vi "Out_S6F11.vi"(8 "error in (no error)":errorcluster, 10 "S6F11":T1, 11 "S6 Message Class in":refnum<class "S6 Message Class.lvclass">) -> (0 "error out":errorcluster, 3 "S6 Message Class out":refnum<class "S6 Message Class.lvclass">)   [LabVIEW 2020, in "SECS Communication.lvlib" / "S6 Message Class.lvclass"]
uses:
  S6 Message Class.lvclass
  D:/Dropbox/SECS/SECS_GEM v1.0.6/Com/SECS Communication/SECS-II Class/SECS-II Class.lvclass
  S6F11.ctl
  SECS-II Class/Format Code.ctl
  SECS-II Class/Data Message_List.vi
  SECS-II Class/Data Message_U4.vi
  SECS-II Class/Variant To Data_ASCII.vi
  SECS-II Class/Data Message_ASCII.vi
  SECS-II Class/Variant To Data_Binary.vi
  SECS-II Class/Data Message_Binary.vi
  SECS-II Class/Variant To Data_Boolean.vi
  SECS-II Class/Data Message_Boolean.vi
  SECS-II Class/Variant To Data_J.vi
  SECS-II Class/Data Message_J.vi
  SECS-II Class/Variant To Data_I1.vi
  SECS-II Class/Data Message_I1 .vi
  SECS-II Class/Variant To Data_I2.vi
  SECS-II Class/Data Message_I2.vi
  SECS-II Class/Variant To Data_I4.vi
  SECS-II Class/Data Message_I4.vi
  SECS-II Class/Variant To Data_I8.vi
  SECS-II Class/Data Message_I8.vi
  SECS-II Class/Variant To Data_U1.vi
  SECS-II Class/Data Message_U1.vi
  SECS-II Class/Variant To Data_U2.vi
  SECS-II Class/Data Message_U2.vi
  SECS-II Class/Variant To Data_U4.vi
  SECS-II Class/Variant To Data_U8.vi
  SECS-II Class/Data Message_U8.vi
  SECS-II Class/Variant To Data_F4.vi
  SECS-II Class/Data Message_F4.vi
  SECS-II Class/Variant To Data_F8.vi
  SECS-II Class/Data Message_F8.vi
  SECS-II Class/Variant To Data_Character.vi
  SECS-II Class/Data Message_Character.vi
  SECS-II Class/SECS-II Class.lvclass
  D:/Dropbox/SECS/SECS_GEM v1.0.6/Com/SECS Communication/S6 Message Class/S6 Message Class.lvclass
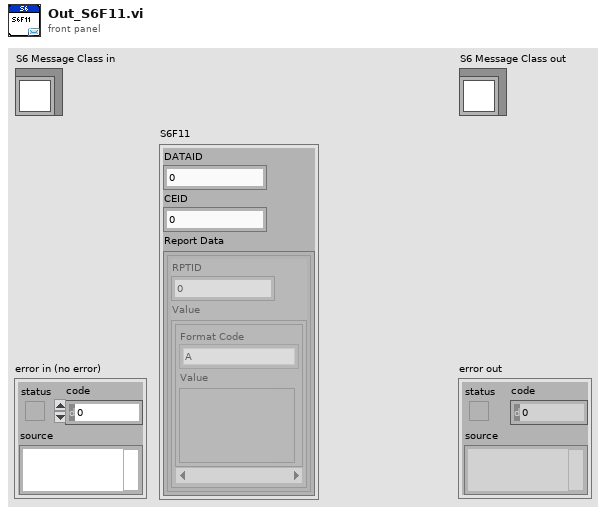
[diagram p1: front panel]
types:
  T1 = typedef "SECS Communication.lvlib/S6 Message Class.lvclass/S6F11.ctl" = cluster{"DATAID":u32, "CEID":u32, "Report Data":cluster{"RPTID":u32, "Value":cluster{"Format Code":T2, "Value":variant}[]}[]}
  T2 = typedef "SECS Communication.lvlib/SECS-II Class.lvclass/Format Code.ctl" = enum16{"L", "A", "B", "Boolean", "J", "I1", "I2", "I4", "I8", "U1", "U2", "U4", "U8", "F4", "F8", "Char"}
  T3 = cluster{"RPTID":u32, "Value":cluster{"Format Code":T2, "Value":variant}[]}[]
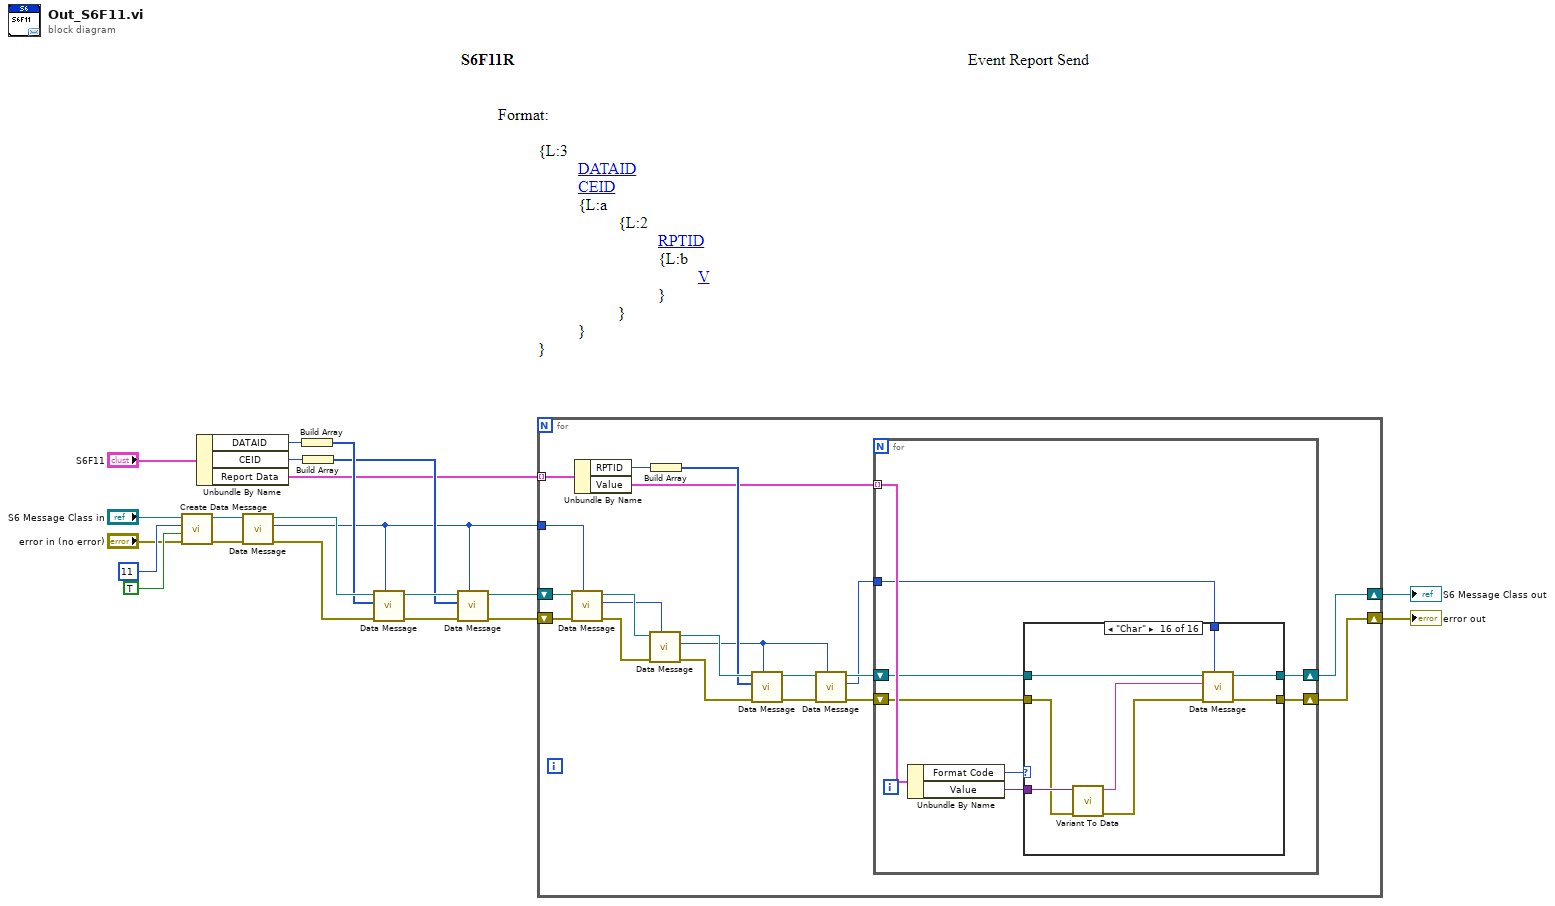
[diagram p0: block diagram]
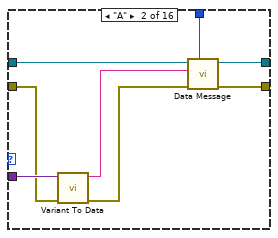
[diagram p3: hidden frame]
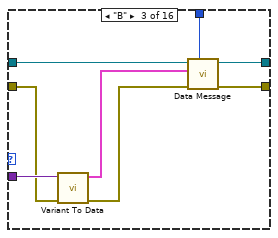
[diagram p4: hidden frame]
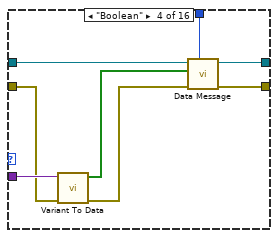
[diagram p5: hidden frame]
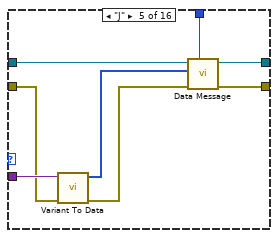
[diagram p6: hidden frame]
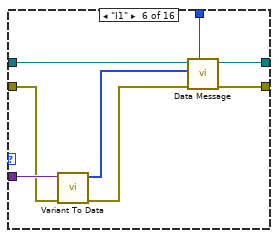
[diagram p7: hidden frame]
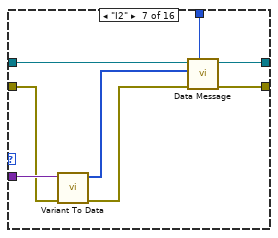
[diagram p8: hidden frame]
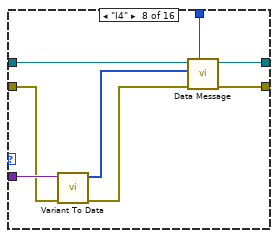
[diagram p9: hidden frame]
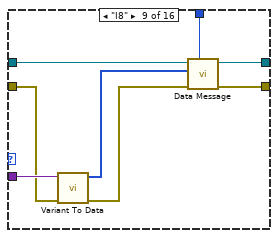
[diagram p10: hidden frame]
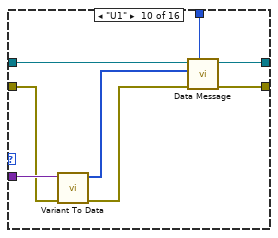
[diagram p11: hidden frame]
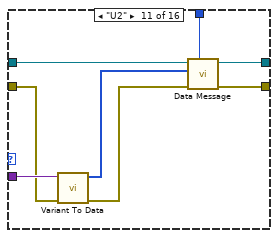
[diagram p12: hidden frame]
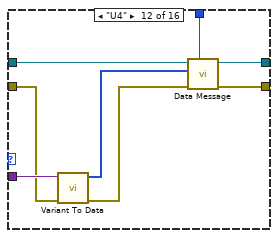
[diagram p13: hidden frame]
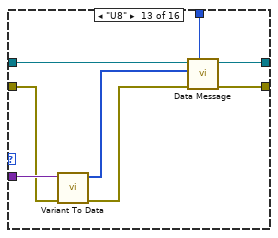
[diagram p14: hidden frame]
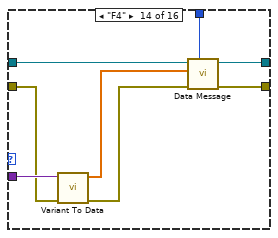
[diagram p15: hidden frame]
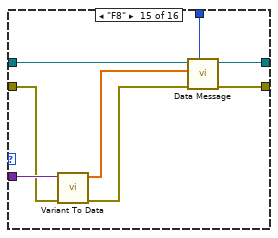
[diagram p16: hidden frame]
diagram:
  n1 = call "Create Data Message.vi"("error in (no error)"="error in (no error)", "W-Bit"=TRUE, "Function"=u8 11, "SECS-II Class in"="S6 Message Class in") -> ("error out"=w18:errorcluster, "SECS-II Class out"=w19:refnum<class "S6 Message Class.lvclass">)  [unwired: 6 in]
  n2 = Unbundle By Name("S6F11") -> ("DATAID"=w12:u32, "CEID"=w8:u32, "Report Data"=w3:T3)
  n3 = call-poly "Data Message.vi"("error in"=w18, "SECS-II Class in"=w19) -> ("error out"=w13:errorcluster, "Index"=w4:i32, "SECS-II Class out"=w14:refnum<class "S6 Message Class.lvclass">)  [unwired: 7 in]
  n4 = Build Array(w12) -> (w11:u32[])
  n5 = Build Array(w8) -> (w7:u32[])
  n6 = call-poly "Data Message.vi"("Parent Index"=w4, "error in"=w13, "Data"=w11, "SECS-II Class in"=w14) -> ("error out"=w9:errorcluster, "SECS-II Class out"=w10:refnum<class "S6 Message Class.lvclass">)  [unwired: 6 in]
  n7 = call-poly "Data Message.vi"("Parent Index"=w4, "error in"=w9, "Data"=w7, "SECS-II Class in"=w10) -> ("error out"=w5:errorcluster, "SECS-II Class out"=w6:refnum<class "S6 Message Class.lvclass">)  [unwired: 6 in]
  n8 = for {
    shift-right: [w22] -> w1
    shift-left: w5 -> [w41]
    shift-right: [w23] -> w2
    shift-left: w6 -> [w40]
    tunnel: w4 -> [w39]
    tunnel: w3 -> [w35] mode=indexing
    n9 = call-poly "Data Message.vi"("Parent Index"=w39, "error in"=w41, "SECS-II Class in"=w40) -> ("error out"=w38:errorcluster, "Index"=w36:i32, "SECS-II Class out"=w37:refnum<class "S6 Message Class.lvclass">)  [unwired: 6 in]
    n10 = Unbundle By Name(w35) -> ("RPTID"=w32:u32, "Value"=w30:cluster{"Format Code":T2, "Value":variant}[])
    n11 = call-poly "Data Message.vi"("Parent Index"=w36, "error in"=w38, "SECS-II Class in"=w37) -> ("error out"=w34:errorcluster, "Index"=w26:i32, "SECS-II Class out"=w33:refnum<class "S6 Message Class.lvclass">)  [unwired: 6 in]
    n12 = Build Array(w32) -> (w31:u32[])
    n13 = call-poly "Data Message.vi"("Parent Index"=w26, "error in"=w34, "Data"=w31, "SECS-II Class in"=w33) -> ("error out"=w27:errorcluster, "SECS-II Class out"=w28:refnum<class "S6 Message Class.lvclass">)  [unwired: 6 in]
    n14 = call-poly "Data Message.vi"("Parent Index"=w26, "error in"=w27, "SECS-II Class in"=w28) -> ("error out"=w25:errorcluster, "Index"=w24:i32, "SECS-II Class out"=w29:refnum<class "S6 Message Class.lvclass">)  [unwired: 6 in]
    n15 = for {
      shift-right: [w44] -> w23
      shift-left: w29 -> [w47]
      shift-right: [w43] -> w22
      shift-left: w25 -> [w48]
      tunnel: w30 -> [w49] mode=indexing
      tunnel: w24 -> [w42]
      n16 = Unbundle By Name(w49) -> ("Format Code"=w46:T2, "Value"=w45:variant)
      n17 = case shown="\"Char\"" w46 {
        tunnel: w45 -> [_ w55 w63 w71 w79 w87 w95 w103 w111 w119 w127 w135 w143 w151 w159 w167]
        tunnel: w47 -> [w51 w59 w67 w75 w83 w91 w99 w107 w115 w123 w131 w139 w147 w155 w163 w171]
        tunnel: w48 -> [w50 w54 w62 w70 w78 w86 w94 w102 w110 w118 w126 w134 w142 w150 w158 w166]
        tunnel: [w51 w57 w65 w73 w81 w89 w97 w105 w113 w121 w129 w137 w145 w153 w161 w169] -> w44
        tunnel: [w50 w56 w64 w72 w80 w88 w96 w104 w112 w120 w128 w136 w144 w152 w160 w168] -> w43
        tunnel: w42 -> [_ w58 w66 w74 w82 w90 w98 w106 w114 w122 w130 w138 w146 w154 w162 w170]
        frame "L", Default {
        }
        frame "A" {
          n18 = call-poly "Variant To Data.vi"("error in (no error)"=w54, "Variant"=w55) -> ("error out"=w53:errorcluster, "Data"=w52:string)  [unwired: 7 in, 1 out]
          n19 = call-poly "Data Message.vi"("Parent Index"=w58, "error in"=w53, "Data"=w52, "SECS-II Class in"=w59) -> ("error out"=w56:errorcluster, "SECS-II Class out"=w57:refnum<class "S6 Message Class.lvclass">)  [unwired: 6 in]
        }
        frame "B" {
          n20 = call-poly "Variant To Data.vi"("error in (no error)"=w62, "Variant"=w63) -> ("error out"=w61:errorcluster, "Data Cluster"=w60:cluster{"Data":bool[]}[])  [unwired: 7 in, 1 out]
          n21 = call-poly "Data Message.vi"("Parent Index"=w66, "error in"=w61, "Data Cluster"=w60, "SECS-II Class in"=w67) -> ("error out"=w64:errorcluster, "SECS-II Class out"=w65:refnum<class "S6 Message Class.lvclass">)  [unwired: 6 in]
        }
        frame "Boolean" {
          n22 = call-poly "Variant To Data.vi"("error in (no error)"=w70, "Variant"=w71) -> ("error out"=w69:errorcluster, "Data"=w68:bool[])  [unwired: 7 in, 1 out]
          n23 = call-poly "Data Message.vi"("Parent Index"=w74, "error in"=w69, "Data"=w68, "SECS-II Class in"=w75) -> ("error out"=w72:errorcluster, "SECS-II Class out"=w73:refnum<class "S6 Message Class.lvclass">)  [unwired: 6 in]
        }
        frame "J" {
          n24 = call-poly "Variant To Data.vi"("error in (no error)"=w78, "Variant"=w79) -> ("error out"=w77:errorcluster, "Data"=w76:i64[])  [unwired: 7 in, 1 out]
          n25 = call-poly "Data Message.vi"("Parent Index"=w82, "error in"=w77, "Data"=w76, "SECS-II Class in"=w83) -> ("error out"=w80:errorcluster, "SECS-II Class out"=w81:refnum<class "S6 Message Class.lvclass">)  [unwired: 6 in]
        }
        frame "I1" {
          n26 = call-poly "Variant To Data.vi"("error in (no error)"=w86, "Variant"=w87) -> ("error out"=w85:errorcluster, "Data"=w84:i8[])  [unwired: 7 in, 1 out]
          n27 = call-poly "Data Message.vi"("Parent Index"=w90, "error in"=w85, "Data"=w84, "SECS-II Class in"=w91) -> ("error out"=w88:errorcluster, "SECS-II Class out"=w89:refnum<class "S6 Message Class.lvclass">)  [unwired: 6 in]
        }
        frame "I2" {
          n28 = call-poly "Variant To Data.vi"("error in (no error)"=w94, "Variant"=w95) -> ("error out"=w93:errorcluster, "Data"=w92:i16[])  [unwired: 7 in, 1 out]
          n29 = call-poly "Data Message.vi"("Parent Index"=w98, "error in"=w93, "Data"=w92, "SECS-II Class in"=w99) -> ("error out"=w96:errorcluster, "SECS-II Class out"=w97:refnum<class "S6 Message Class.lvclass">)  [unwired: 6 in]
        }
        frame "I4" {
          n30 = call-poly "Variant To Data.vi"("error in (no error)"=w102, "Variant"=w103) -> ("error out"=w101:errorcluster, "Data"=w100:i32[])  [unwired: 7 in, 1 out]
          n31 = call-poly "Data Message.vi"("Parent Index"=w106, "error in"=w101, "Data"=w100, "SECS-II Class in"=w107) -> ("error out"=w104:errorcluster, "SECS-II Class out"=w105:refnum<class "S6 Message Class.lvclass">)  [unwired: 6 in]
        }
        frame "I8" {
          n32 = call-poly "Variant To Data.vi"("error in (no error)"=w110, "Variant"=w111) -> ("error out"=w109:errorcluster, "Data"=w108:i64[])  [unwired: 7 in, 1 out]
          n33 = call-poly "Data Message.vi"("Parent Index"=w114, "error in"=w109, "Data"=w108, "SECS-II Class in"=w115) -> ("error out"=w112:errorcluster, "SECS-II Class out"=w113:refnum<class "S6 Message Class.lvclass">)  [unwired: 6 in]
        }
        frame "U1" {
          n34 = call-poly "Variant To Data.vi"("error in (no error)"=w118, "Variant"=w119) -> ("error out"=w117:errorcluster, "Data"=w116:u8[])  [unwired: 7 in, 1 out]
          n35 = call-poly "Data Message.vi"("Parent Index"=w122, "error in"=w117, "Data"=w116, "SECS-II Class in"=w123) -> ("error out"=w120:errorcluster, "SECS-II Class out"=w121:refnum<class "S6 Message Class.lvclass">)  [unwired: 6 in]
        }
        frame "U2" {
          n36 = call-poly "Variant To Data.vi"("error in (no error)"=w126, "Variant"=w127) -> ("error out"=w125:errorcluster, "Data"=w124:u16[])  [unwired: 7 in, 1 out]
          n37 = call-poly "Data Message.vi"("Parent Index"=w130, "error in"=w125, "Data"=w124, "SECS-II Class in"=w131) -> ("error out"=w128:errorcluster, "SECS-II Class out"=w129:refnum<class "S6 Message Class.lvclass">)  [unwired: 6 in]
        }
        frame "U4" {
          n38 = call-poly "Variant To Data.vi"("error in (no error)"=w134, "Variant"=w135) -> ("error out"=w133:errorcluster, "Data"=w132:u32[])  [unwired: 7 in, 1 out]
          n39 = call-poly "Data Message.vi"("Parent Index"=w138, "error in"=w133, "Data"=w132, "SECS-II Class in"=w139) -> ("error out"=w136:errorcluster, "SECS-II Class out"=w137:refnum<class "S6 Message Class.lvclass">)  [unwired: 6 in]
        }
        frame "U8" {
          n40 = call-poly "Variant To Data.vi"("error in (no error)"=w142, "Variant"=w143) -> ("error out"=w141:errorcluster, "Data"=w140:u64[])  [unwired: 7 in, 1 out]
          n41 = call-poly "Data Message.vi"("Parent Index"=w146, "error in"=w141, "Data"=w140, "SECS-II Class in"=w147) -> ("error out"=w144:errorcluster, "SECS-II Class out"=w145:refnum<class "S6 Message Class.lvclass">)  [unwired: 6 in]
        }
        frame "F4" {
          n42 = call-poly "Variant To Data.vi"("error in (no error)"=w150, "Variant"=w151) -> ("error out"=w149:errorcluster, "Data"=w148:sgl[])  [unwired: 7 in, 1 out]
          n43 = call-poly "Data Message.vi"("Parent Index"=w154, "error in"=w149, "Data"=w148, "SECS-II Class in"=w155) -> ("error out"=w152:errorcluster, "SECS-II Class out"=w153:refnum<class "S6 Message Class.lvclass">)  [unwired: 6 in]
        }
        frame "F8" {
          n44 = call-poly "Variant To Data.vi"("error in (no error)"=w158, "Variant"=w159) -> ("error out"=w157:errorcluster, "Data"=w156:dbl[])  [unwired: 7 in, 1 out]
          n45 = call-poly "Data Message.vi"("Parent Index"=w162, "error in"=w157, "Data"=w156, "SECS-II Class in"=w163) -> ("error out"=w160:errorcluster, "SECS-II Class out"=w161:refnum<class "S6 Message Class.lvclass">)  [unwired: 6 in]
        }
        frame "Char" {
          n46 = call-poly "Variant To Data.vi"("error in (no error)"=w166, "Variant"=w167) -> ("error out"=w165:errorcluster, "Data"=w164:string)  [unwired: 7 in, 1 out]
          n47 = call-poly "Data Message.vi"("Parent Index"=w170, "error in"=w165, "Data"=w164, "SECS-II Class in"=w171) -> ("error out"=w168:errorcluster, "SECS-II Class out"=w169:refnum<class "S6 Message Class.lvclass">)  [unwired: 6 in]
        }
      }
    }
  }
  "error out" <- w1
  "S6 Message Class out" <- w2
